vi "Test Customer Pick Up Order Broadcasts State.vi"(8 "error in (no error)":errorcluster, 11 "Customer Test in":refnum<class "Customer Test.lvclass">) -> (0 "error out":errorcluster, 3 "Customer Test out":refnum<class "Customer Test.lvclass">)   [LabVIEW 2020, in "Customer Test.lvclass"]
uses:
  Customer Test.lvclass
  C:/Program Files (x86)/National Instruments/LabVIEW 2020/vi.lib/Asteme/LUnit/Test Case.lvclass
  Processes/People/Customers/Customer/Customer.lvclass
  C:/Program Files (x86)/National Instruments/LabVIEW 2020/vi.lib/Asteme/Triarc Framework/Process/Process.lvclass
  Support/Beverages/Beverage/Beverage.lvclass
  Processes/People/Customers/Customer/Public/Order State.ctl
  <vilib>/Asteme/Triarc Framework/Process/Process.lvclass/Process.ctl
  <vilib>/Asteme/LUnit/Test Case.lvclass/Test Case.ctl
  <vilib>/Asteme/LUnit/LUnit Assertion Result.lvclass/LUnit Assertion Result.ctl
  <vilib>/Asteme/Triarc Framework Test Suite/Support/Execution timer.vi
  <vilib>/Asteme/Triarc Framework/Process/Private/SubVIs/Wait for finish.vi
  <vilib>/Asteme/Triarc Framework/Process/Protected/Messaging/Enqueue Message.vi
  <vilib>/Asteme/Triarc Framework/Process/Private/SubVIs/Set Lifecycle State.vi
  <vilib>/Asteme/Triarc Framework/Process/Public/Lifecycle/Get Lifecycle State.vi
  <vilib>/Asteme/LUnit/Palette/Fail.vi
  <vilib>/Asteme/LUnit/Palette/Pass.vi
  <vilib>/Asteme/LUnit/Set Assertion Type.vi
  <vilib>/AdvancedString/1D String Array to Delimited String.vi
  <vilib>/Utility/error.llb/Clear Errors.vi
  <vilib>/Asteme/LUnit/Add test result.vi
  <vilib>/Asteme/LUnit/LUnit Write Passed.vi
  <vilib>/Asteme/LUnit/LUnit Get Test Case.vi
  <vilib>/Asteme/LUnit/Assertion Result/LUnit Get Test Name.vi
  <vilib>/Asteme/LUnit/LUnit Write Message.vi
  <vilib>/Asteme/LUnit/LUnit Write Description.vi
  <vilib>/Asteme/LUnit/LUnit Write Assertion Type.vi
  <vilib>/Asteme/LUnit/Read Test Case Name.vi
  <vilib>/Asteme/Triarc Framework Test Suite/Support/Event Helpers/Dequeue Event Message.vi
  <vilib>/Utility/error.llb/Error Cluster From Error Code.vi
  <vilib>/Asteme/LUnit/LUnit Assertion Result.lvclass
  <vilib>/Asteme/Triarc Framework/Process/Process.lvclass
  <vilib>/Asteme/Triarc Framework Test Suite/Support/Event Helpers/Event Helpers.lvlib
  <vilib>/Asteme/LUnit/Test Case.lvclass
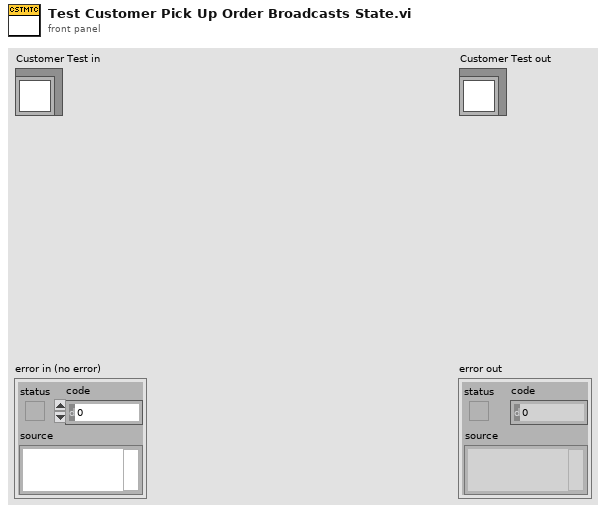
[diagram p1: front panel]
types:
  T1 = typedef "Customer.lvclass/Order State.ctl" = cluster{"Order In Progress?":bool, "Order Number":u32, "Order Price":dbl, "Items Ordered":u32, "Items Received":u32, "Items Picked Up":string}
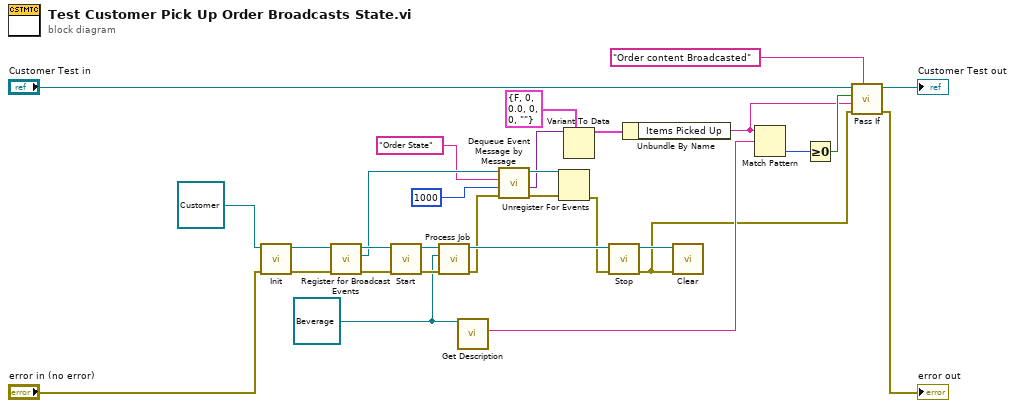
[diagram p0: block diagram]
diagram:
  w8 = refnum<class "Beverage.lvclass"> refnum ("Beverage.lvclass")
  n1 = call-dynamic "Init.vi"("error in (no error)"="error in (no error)", "View In"=refnum<class "Customer.lvclass"> refnum ("Customer.lvclass")) -> ("error out"=w26:errorcluster, "View Out"=w27:refnum<class "Customer.lvclass">)  [unwired: 8 in]
  n2 = call <vilib>:"Register for Broadcast Events.vi"("error in (no error)"=w26, "Process In"=w27) -> ("error out"=w29:errorcluster, "Event Registration Refnum Out"=w23:refnum<event-registration>, "Process Out"=w28:refnum<class "Customer.lvclass">)  [unwired: 7 in]
  n3 = call <vilib>:"Start.vi"("error in (no error)"=w29, "Process In"=w28) -> ("error out"=w20:errorcluster, "Process Out"=w22:refnum<class "Customer.lvclass">)  [unwired: 8 in]
  n4 = call-dynamic "Process Job.vi"("error in (no error)"=w20, "Job"=w8, "Process Job In"=w22) -> ("error out"=w19:errorcluster, "Process Job Out"=w21:refnum<class "Customer.lvclass">)  [unwired: 7 in]
  n5 = call "Get Description.vi"("Beverage in"=w8) -> ("Description"=w5:string)  [unwired: 8 in, 2 out]
  n6 = call <vilib>:"Dequeue Event Message by Message.vi"("error in (no error)"=w19, "Timeout (-1)"=1000, "Message"="Order State", "Event Registration Refnum"=w23) -> ("error out"=w18:errorcluster, "Message Data"=w9:variant, "Event Registration Refnum Out"=w12:refnum<event-registration>)  [unwired: 3 in, 2 out]
  n7 = Unregister For Events(event registration refnum=w12, error in=w18) -> (error out=w15:errorcluster)
  n8 = Variant To Data(type=T1 {"Order In Progress?"=FALSE, "Order Number"=0, "Order Price"=0.0, "Items Ordered"=0, "Items Received"=0, "Items Picked Up"=""} ("Order State"), Variant=w9) -> (data=w6:T1)  [unwired: 1 in, 1 out]
  n9 = call <vilib>:"Stop.vi"("error in (no error)"=w15, "Process In"=w21) -> ("error out"=w1:errorcluster, "Process Out"=w25:refnum<class "Customer.lvclass">)  [unwired: 7 in, 1 out]
  n10 = Unbundle By Name(w6) -> ("Items Picked Up"=w2:string)
  n11 = call-dynamic "Clear.vi"("error in (no error)"=w1, "View In"=w25) -> ()  [unwired: 9 in, 1 out]
  n12 = Match Pattern(string=w2, regular expression=w5) -> (offset past match=w4:i32)  [unwired: 1 in, 3 out]
  n13 = Greater Or Equal To 0?(x=w4) -> (x >= 0?=w3:bool)
  n14 = call <vilib>:"Pass If.vi"("Description"="Order content Broadcasted", "error in (no error)"=w1, "Message"=w2, "Pass?"=w3, "Test Case In"="Customer Test in") -> ("error out"=→"error out":errorcluster, "Test Case Out"=→"Customer Test out":refnum<class "Customer Test.lvclass">)  [unwired: 5 in]
